vi "2_VisualAD_Inference(Image).vi"() -> ()   [LabVIEW 2024]
uses:
  <vilib>/ptbypt/NI_PtbyPt.lvlib
  <vilib>/Ngene/DeepLTK Anomaly Detection Addon/DeepLTK_Anomaly_Detection_Addon/DeepLTK_Anomaly_Detection_Addon.lvlib
  <vilib>/Ngene/Deep Learning Toolkit/Toolkit/NN_Data/API/NN_Dims(C,H,W).ctl
  <vilib>/Ngene/Deep Learning Toolkit/Toolkit/Deep_Learning_Toolkit_by_Ngene.lvlib
  <vilib>/Ngene/Deep Learning Toolkit/Toolkit/NN_Network/Controls/NN_Device.ctl
  subVIs/Visualizer/Controls/ROI_Display_Options.ctl
  subVIs/Visualizer/Controls/ColorMap.ctl
  subVIs/Visualizer/Controls/Heatmap_Display_Options.ctl
  subVIs/Visualizer/Controls/Display_Options.ctl
  <vilib>/Ngene/DeepLTK Anomaly Detection Addon/DeepLTK_Anomaly_Detection_Addon/API/Controls/Gaussian_Blur.ctl
  <vilib>/Ngene/DeepLTK Anomaly Detection Addon/DeepLTK_Anomaly_Detection_Addon/API/Controls/Feature_Scorer_Params.ctl
  <vilib>/Ngene/DeepLTK Anomaly Detection Addon/DeepLTK_Anomaly_Detection_Addon/API/Controls/NN_Paths.ctl
  <vilib>/Ngene/DeepLTK Anomaly Detection Addon/DeepLTK_Anomaly_Detection_Addon/API/Controls/NNPC_Setup.ctl
  <vilib>/Ngene/DeepLTK Anomaly Detection Addon/DeepLTK_Anomaly_Detection_Addon/API/Controls/MinMax.ctl
panel:
  in  "Display_Options":T1={"ROI_Options"={"Color"=16711680, "Width"=1, "Drawing Mode"=enum."Frame"}, "Heatmap_Options"={"ColorMap"=enum."Jet", "Alpha"=0.4, "Heatmap Range"={"Min"=1.3, "Max"=-1.0}}, "Has GT?"=FALSE} {"Heatmap_Options"."Heatmap Range"."Min" format="%#_5g"}
  out "dT_Init":dbl=0.2686297510000486 format="%#_3ps"
  in  "NNPC_Paths":T6={"CFG"=path "D:/Ngene/Projects_SVN/AD/Projects/2025/2025_04_09_VAD_RT_NIConnect/Models/NNPC_RN18_2_bnMerge_LIdx8_HW256_CS1200_PS5__25_04_04__17_31_52/NNPC_RN18_2_bnMerge_LIdx8_HW256_CS1200_PS5.cfg", "BIN"=path "D:/Ngene/Projects_SVN/AD/Projects/2025/2025_04_09_VAD_RT_NIConnect/Models/NNPC_RN18_2_bnMerge_LIdx8_HW256_CS1200_PS5__25_04_04__17_31_52/NNPC_RN18_2_bnMerge_LIdx8_HW256_CS1200_PS5.bin"}
  out "Image_Thrshld (Eval)":sgl=7.5923
  in  "Image_Thrshld(Custom)":sgl=-1.0 format="%_5g"
  out "dT_Predict":dbl=0.6672163729800036 format="%#_3ps"
  out "Pixel_Score(Min)":sgl=0.8570011
  out "Pixel_Score(Max)":sgl=6.2930846
  out "Image_File_Path":path=path "D:/Cards_v2/Test/good/ (1).bmp"
  in  "Feature_Scorer_Params":T7={"Nearest_Neighbors"=1, "Calculate Anomaly Map"=TRUE, "Gaussian_Blur"={"Kernel_Size"=33, "Sigma"=4.0}}
  out "Pixel_Thrshld (Eval)":sgl=1.1519
  in  "Stop":bool
  out "Anomaly?":bool
  out "dT_ImRead":dbl=0.020058404999986124 format="%#_4ps"
  in  "NNPC_Setup":T9={"Input_Dims"={"C"=-1, "H"=-1, "W"=-1}, "mBatch"=1, "Device"=enum."CPU", "GPU Id"=0}
  out "Anomaly Detection Results":T12(plugin-control)
  out "Img_Score":sgl=7.444628
  in  "Image_idx":u32 max=248
  in  "Ground_Truth_Folder_Path":path
  in  "Pixel_Thrshld(Custom)":sgl=7.0 format="%_5g"
  in  "Test_Dataset_Folder_Path":path=path "D:/Cards_v2/Test"
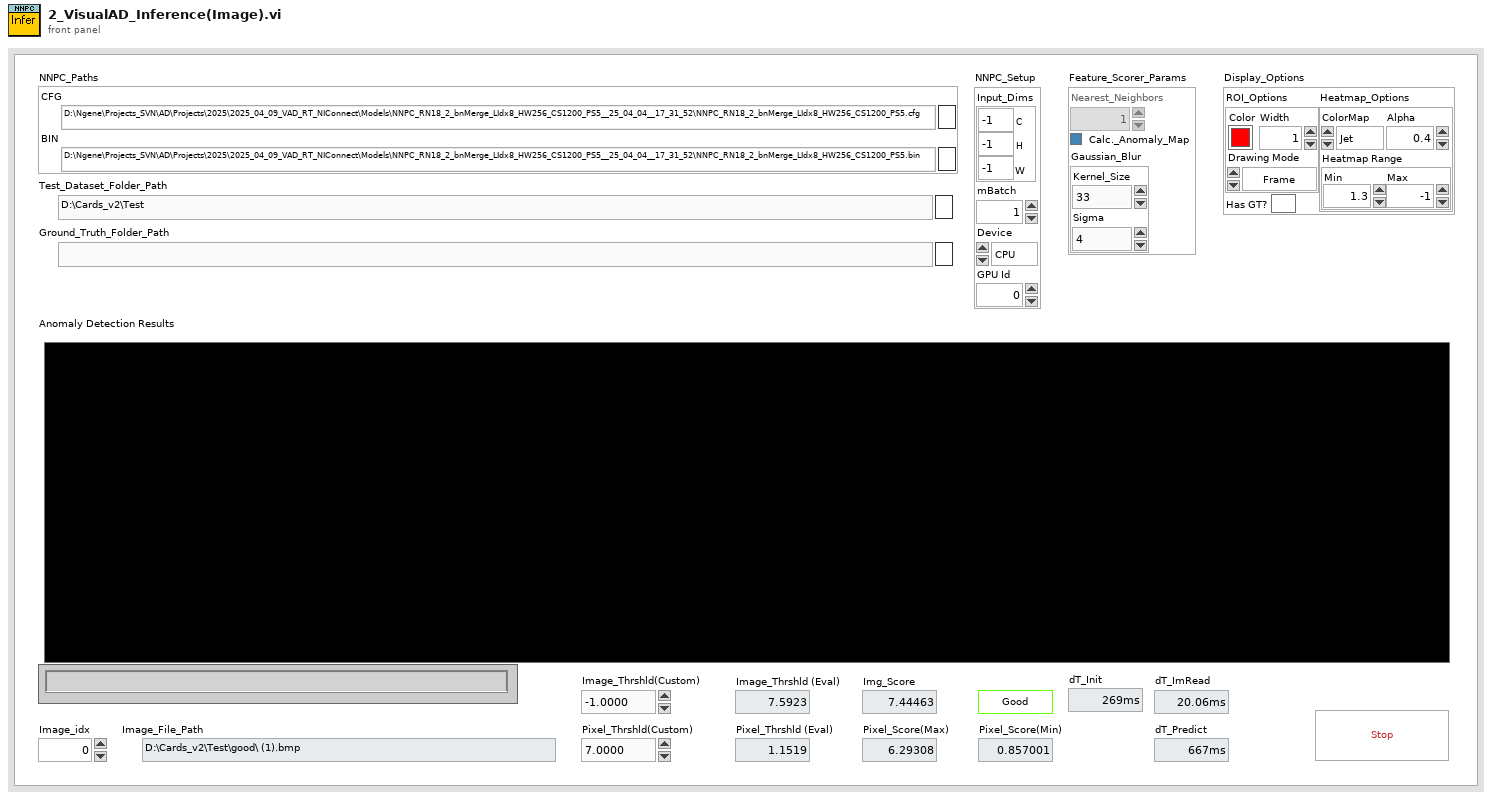
[diagram p1: front panel]
types:
  T1 = typedef "Display_Options.ctl" = cluster{"ROI_Options":T2, "Heatmap_Options":T3, "Has GT?":bool}
  T2 = typedef "ROI_Display_Options.ctl" = cluster{"Color":u32, "Width":u32, "Drawing Mode":enum16{"Frame", "Fill"}}
  T3 = typedef "Heatmap_Display_Options.ctl" = cluster{"ColorMap":T4, "Alpha":sgl, "Heatmap Range":T5}
  T4 = typedef "ColorMap.ctl" = enum16{"Jet", "Perula", "Inferno", "Plasma", "Viridis"}
  T5 = typedef "DeepLTK_Anomaly_Detection_Addon.lvlib/MinMax.ctl" = cluster{"Min":sgl, "Max":sgl}
  T6 = typedef "DeepLTK_Anomaly_Detection_Addon.lvlib/NN_Paths.ctl" = cluster{"CFG":path, "BIN":path}
  T7 = typedef "DeepLTK_Anomaly_Detection_Addon.lvlib/Feature_Scorer_Params.ctl" = cluster{"Nearest_Neighbors":i32, "Calculate Anomaly Map":bool, "Gaussian_Blur":T8}
  T8 = typedef "DeepLTK_Anomaly_Detection_Addon.lvlib/Gaussian_Blur.ctl" = cluster{"Kernel_Size":i32, "Sigma":sgl}
  T9 = typedef "DeepLTK_Anomaly_Detection_Addon.lvlib/NNPC_Setup.ctl" = cluster{"Input_Dims":T10, "mBatch":i32, "Device":T11, "GPU Id":i32}
  T10 = typedef "Deep_Learning_Toolkit_by_Ngene.lvlib/NN_Dims(C,H,W).ctl" = cluster{"C":i32, "H":i32, "W":i32}
  T11 = typedef "Deep_Learning_Toolkit_by_Ngene.lvlib/NN_Device.ctl" = enum16{"CPU", "GPU"}
  T12 = typedef "IMAQ Image.ctl" = refnum<image>
  T13 = typedef "DeepLTK_Anomaly_Detection_Addon.lvlib/NNPC_Evaluation_Results.ctl" = cluster{"Threshold(Image)":sgl, "Threshold(Pixel)":sgl, "Pixel_Range":cluster{"Min":sgl, "Max":sgl}}
  T14 = typedef "DeepLTK_Anomaly_Detection_Addon.lvlib/NNPC_PreProcessing_Options.ctl" = cluster{"DS_Name":string, "Input_Dims":T10, "Center Crop Size":i32, "Interpolation Type":u32, "Multi-Stage_DownSample?":bool, "Dataset_Stats":T15}
  T15 = typedef "DeepLTK_Anomaly_Detection_Addon.lvlib/NNPC_DS_Stats.ctl" = cluster{"means":T16, "stds":T16}
  T16 = typedef "DeepLTK_Anomaly_Detection_Addon.lvlib/Image_Stats_RGB.ctl" = cluster{"R":sgl, "G":sgl, "B":sgl}
  T17 = typedef "DeepLTK_Anomaly_Detection_Addon.lvlib/NNPC_Instance.ctl" = cluster{"NN out":T18, "MemBank_Data":T33, "Name":string}
  T18 = typedef "Deep_Learning_Toolkit_by_Ngene.lvlib/NN.ctl" = cluster{"Name":string, "No of Layers":i32, "mBatch":i32, "Layers":T19[], "Dimty":T20, "Dims_In":T10, "Dims_Out":T10, "Working_Dir":path, "Train?":bool, "Train_Params":T21, "LR_Update_Policy":T24, "Session Data":T26, "Ground_truth":T27, "NNg_hdls":T28, "NN_Device":T11, "GPU Id":i32, "Labels":string[], "Receptive Field":T29[], "Loss_Type":T30, "Loss_Cfg_Prms":variant, "NNG_WS":T31}
  T19 = typedef "Deep_Learning_Toolkit_by_Ngene.lvlib/NN_Layer_ref.ctl" = refnum<data-value>
  T20 = typedef "Deep_Learning_Toolkit_by_Ngene.lvlib/NN_In_Out_Dim-ty.ctl" = enum8{"In1D_Out1D", "In3D_Out1D", "In3D_Out3D", "In3D_OutBBox"}
  T21 = typedef "Deep_Learning_Toolkit_by_Ngene.lvlib/NN_Train_Params.ctl" = cluster{"Optimizer":T22, "Beta_1":sgl, "Beta_2":sgl, "Weight Decay(L1)":sgl, "Weight Decay(L2)":sgl, "Data_Sampling":T23}
  T22 = typedef "Deep_Learning_Toolkit_by_Ngene.lvlib/NN_Train_Optimizer.ctl" = enum16{"SGD", "Adam", "Adagrad", "Adadelta", "RMSProp", "Nesterov"}
  T23 = typedef "Deep_Learning_Toolkit_by_Ngene.lvlib/NN_Train_Data_Sampling.ctl" = enum16{"Random", "Sequential"}
  T24 = typedef "Deep_Learning_Toolkit_by_Ngene.lvlib/NN_LR_Policy_Cfg.ctl" = cluster{"Policy_Type":T25, "LR0":dbl, "k":sgl, "WarmUp_Policy":enum16{"Step", "Ramp"}, "WarmUp_Iter":i32, "WarmUp_Ratio":sgl}
  T25 = typedef "Deep_Learning_Toolkit_by_Ngene.lvlib/NN_LR_Policy_Type.ctl" = enum16{"Manual", "Step", "Exp", "1/t"}
  T26 = typedef "Deep_Learning_Toolkit_by_Ngene.lvlib/NN_Train_Session_Data.ctl" = cluster{"Epochs":sgl, "Tot_Iter":i32, "LR":sgl, "LR_iter":i32}
  T27 = typedef "Deep_Learning_Toolkit_by_Ngene.lvlib/NN_Ground_truth.ctl" = cluster{"Y":variant}
  T28 = typedef "Deep_Learning_Toolkit_by_Ngene.lvlib/nng_cuda_handles.ctl" = cluster{"cudnn":u64, "cublas":u64, "stream":u64, "curand":u64}
  T29 = typedef "Deep_Learning_Toolkit_by_Ngene.lvlib/NN_Dims(V,H).ctl" = cluster{"V":i32, "H":i32}
  T30 = typedef "Deep_Learning_Toolkit_by_Ngene.lvlib/NN_Loss_Type.ctl" = enum16{"None", "MSE", "CrossEntropy", "YOLO_v2", "YOLO_v4"}
  T31 = typedef "Deep_Learning_Toolkit_by_Ngene.lvlib/NNG_WS.ctl" = cluster{"NNG_WS_Mem":T32, "Max_WS_Size":i64}
  T32 = typedef "Deep_Learning_Toolkit_by_Ngene.lvlib/NNg_WS_Mem_DVR.ctl" = refnum<data-value>
  T33 = typedef "DeepLTK_Anomaly_Detection_Addon.lvlib/MemBank_and_Norm_Variants.ctl" = cluster{"MemBank":variant, "MemBank Norm":variant}
  T34 = typedef "Anomaly_Detection_Results_Imgs.ctl" = cluster{"Image":T12, "Ground Truth":T12, "Predicted Heat Map":T12, "Predicted Mask":T12, "Segmentation":T12}
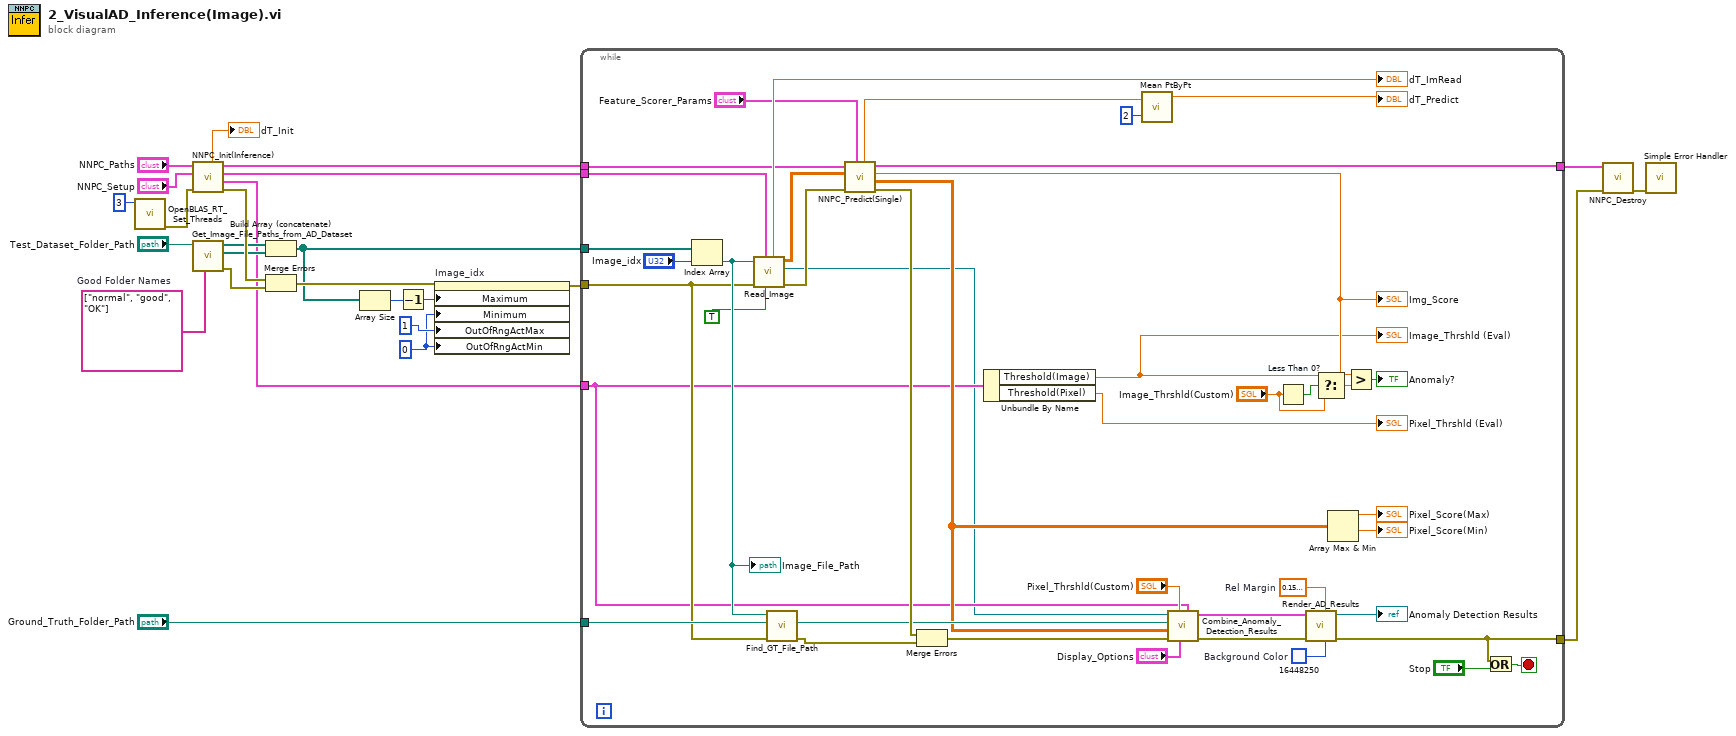
[diagram p0: block diagram]
diagram:
  w4 = string[] ["normal", "good", "OK"]  # Good Folder Names
  w6 = u32 0 ("Data Entry Limits:Minimum")
  n1 = call "OpenBLAS_RT_Set_Threads.vi"("threads"=3) -> ("error out"=w2:errorcluster)  [unwired: 10 in]
  n2 = call <vilib>:"NNPC_Init(Inference).vi"("error in"=w2, "NNPC_Setup"="NNPC_Setup", "NNPC_Paths"="NNPC_Paths") -> ("error out"=w23:errorcluster, "Evaluation_Results"=w7:T13, "PreProc_Options"=w9:T14, "NNPC_out"=w24:T17, "dT_Init_Inference"=→"dT_Init":dbl)  [unwired: 4 in]
  n3 = call "Get_Image_File_Paths_from_AD_Dataset.vi"("Good Folder Names"=w4, "Dataset Folder"="Test_Dataset_Folder_Path") -> ("error out"=w21:errorcluster, "Bad Dataset Files"=w17:path[], "Good Dataset Files"=w16:path[])  [unwired: 7 in]
  n4 = Build Array (concatenate)(w16, w17) -> (w3:path[])
  n5 = Merge Errors(w23, w21) -> (w11:errorcluster)
  n6 = Array Size(array=w3) -> (size(s)=w12:i32)
  n7 = Decrement(x=w12) -> (x-1=w14:i32)
  n8 = property on="Image_idx" class="DigNum (strict)"(error in=w11, "Maximum"=w14, "Minimum"=w6, "OutOfRngActMax"=u8 1 ("Response to Value Outside Limits:Maximum"), "OutOfRngActMin"=w6) -> (error out=w10:errorcluster)  [unwired: 1 in, 1 out]
  n9 = while {
    tunnel: w3 -> [w67]
    tunnel: w24 -> [w49]
    tunnel: [w43] -> w19
    tunnel: w10 -> [w38]
    tunnel: [w40] -> w20
    tunnel: "Ground_Truth_Folder_Path" -> [w52]
    tunnel: w9 -> [w35]
    tunnel: w7 -> [w31]
    stop <- w41 stop-if-true
    w39 = u32 16448250  # Background Color
    w59 = sgl 0.15  # Rel Margin
    n10 = Index Array(array=w67, index="Image_idx") -> (element=w54:path)
    "Image_File_Path" <- w54
    n11 = call "Read_Image.vi"(6:TRUE ("MultyStage_Resample?"), "PreProcessing_Options"=w35, "error in"=w38, "Img Path"=w54) -> ("error out"=w44:errorcluster, "Imaq Image Out"=w30:T12, "Image Out"=w28:sgl[][][], "dT_Img_Read"=→"dT_ImRead":dbl)  [unwired: 4 in]
    n12 = call "Find_GT_File_Path.vi"("error in"=w38, "GT Mask Folder Path"=w52, "Image File Path"=w54) -> ("error out"=w36:errorcluster, "GT File Path"=w53:path)  [unwired: 5 in, 2 out]
    n13 = call <vilib>:"NNPC_Predict(Single).vi"("Feature_Scorer_Params"="Feature_Scorer_Params", "error in"=w44, "Image_in"=w28, "NNPC_in"=w49) -> ("error out"=w65:errorcluster, "Anomaly_Map"=w48:sgl[][], "Pred_Score"=w47:sgl, "NNPC_out"=w43:T17, "dT_Predict"=w34:dbl)  [unwired: 3 in]
    "Img_Score" <- w47
    n14 = Merge Errors(w65, w36) -> (w37:errorcluster)
    n15 = Unbundle By Name(w31) -> ("Threshold(Image)"=w33:sgl, "Threshold(Pixel)"=→"Pixel_Thrshld (Eval)":sgl)
    "Image_Thrshld (Eval)" <- w33
    n16 = call <vilib>:"Mean PtByPt.vi"("x"=w34, "sample length"=2) -> ("mean"=→"dT_Predict":dbl)  [unwired: 2 in, 1 out]
    n17 = call "Combine_Anomaly_Detection_Results.vi"("Evaluation_Results"=w31, "Display_Options"="Display_Options", "Pixel Anomaly Thrshld"="Pixel_Thrshld(Custom)", "error in"=w37, "Anomaly Map"=w48, "Gt File Path"=w53, "Orig Image In"=w30) -> ("error out"=w64:errorcluster, "Anomaly Detection Rresults"=w63:T34)  [unwired: 2 in, 1 out]
    n18 = Less Than 0?(x="Image_Thrshld(Custom)") -> (x < 0?=w58:bool)
    n19 = call "Render_AD_Results.vi"("Background Color"=w39, "Rel._Margin"=w59, "error in"=w64, "Anomaly Detection Rresults"=w63) -> ("error out"=w40:errorcluster, "Anomaly Detection Results"=→"Anomaly Detection Results":T12)  [unwired: 6 in]
    n20 = Select(t=w33, s=w58, f="Image_Thrshld(Custom)") -> (s? t:f=w56:sgl)
    n21 = Array Max & Min(array=w48) -> (max value=→"Pixel_Score(Max)":sgl, min value=→"Pixel_Score(Min)":sgl)  [unwired: 2 out]
    n22 = Greater?(x=w47, y=w56) -> (0:→"Anomaly?":bool)
    n23 = Or(x=w40, y="Stop") -> (x .or. y?=w41:bool)
  }
  n24 = call <vilib>:"NNPC_Destroy.vi"("error in"=w20, "NNPC_in"=w19) -> ("error out"=w18:errorcluster)  [unwired: 9 in]
  n25 = call <vilib>:"Simple Error Handler.vi"("error in (no error)"=w18) -> ()  [unwired: 4 in, 5 out]
